vi "ST5 Move Status.vi"(0 "Port COM":refnum<visa-resource-name>, 1 "Facteur Pas":dbl=1500.0, 2 "Facteur Dir":bool, 5 "Delay(s)":i32=40, 9 "Stop Ref":refnum<vi>, 11 "error in":errorcluster, 12 "Pos Ref":refnum<vi>) -> (4 "Port Out":refnum<visa-resource-name>, 6 "CCW Limit":bool, 8 "Alarme":u32, 10 "CW Limit":bool, 14 "Status":T1, 15 "error out":errorcluster)   [LabVIEW 2019]
panel:
  out "Position":dbl
  in  "Stop":bool
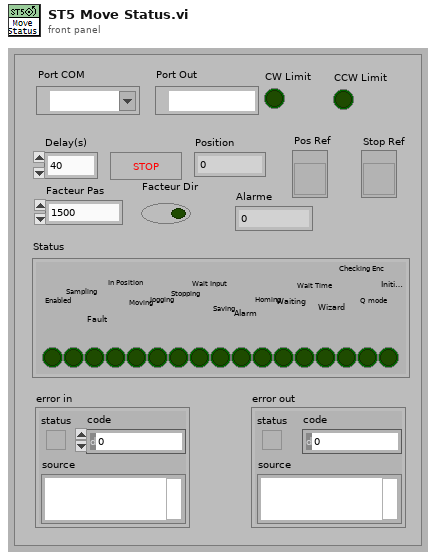
[diagram p1: front panel]
types:
  T1 = cluster{"Enabled":bool, "Sampling":bool, "Fault":bool, "In Position":bool, "Moving":bool, "Jogging":bool, "Stopping":bool, "Wait Input":bool, "Saving":bool, "Alarm":bool, "Homing":bool, "Waiting":bool, "Wait Time":bool, "Wizard":bool, "Checking Enc":bool, "Q mode":bool, "Initializing":bool}
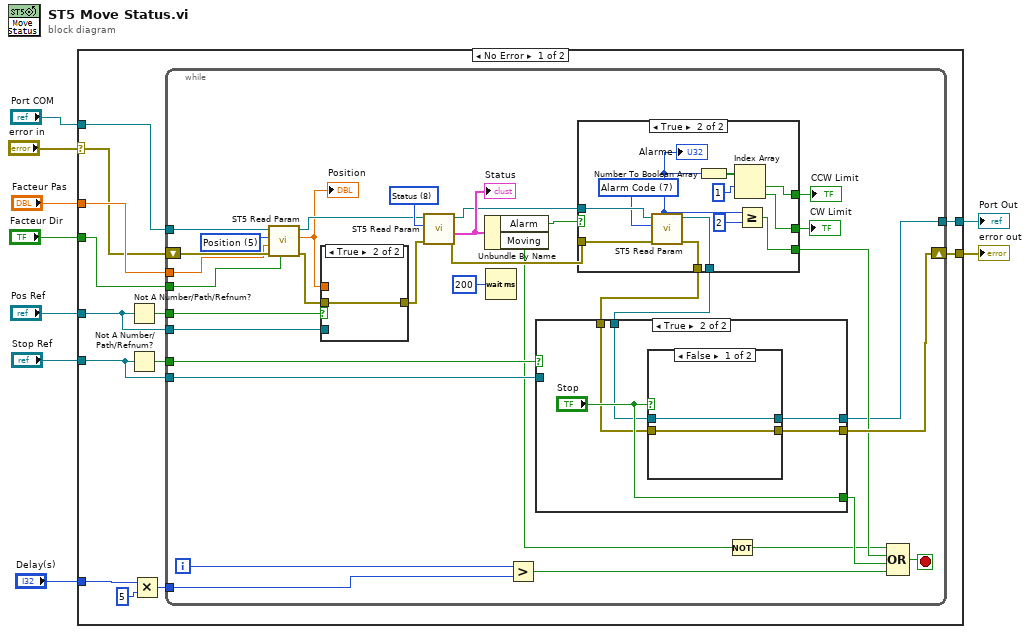
[diagram p0: block diagram]
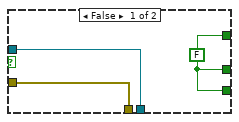
[diagram p2: hidden frame]
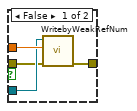
[diagram p3: hidden frame]
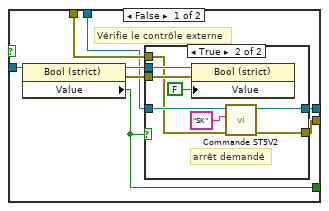
[diagram p4: hidden frame]
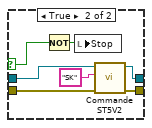
[diagram p6: hidden frame]
diagram:
  n1 = case shown="No Error" "error in" {
    selector: "error in" -> [w12 w109]
    tunnel: [w22 w109] -> w9
    tunnel: "Port COM" -> [w15 w108]
    tunnel: [w21 w108] -> w7
    tunnel: "Delay(s)" -> [w20 _]
    tunnel: "Stop Ref" -> [w16 _]
    tunnel: "Facteur Pas" -> [w14 _]
    tunnel: "Facteur Dir" -> [w13 _]
    tunnel: "Pos Ref" -> [w10 _]
    frame No Error {
      n2 = Not A Number/Path/Refnum?(number/path/refnum=w10) -> (NaN/Path/Refnum?=w11:bool)
      n3 = Not A Number/Path/Refnum?(number/path/refnum=w16) -> (NaN/Path/Refnum?=w17:bool)
      n4 = Multiply(x=w20, y=5) -> (x*y=w18:i32)
      n5 = while {
        tunnel: w15 -> [w46]
        shift-right: [w45] -> w22
        shift-left: w12 -> [w53]
        tunnel: [w25] -> w21
        tunnel: w18 -> [w52]
        tunnel: w17 -> [w50]
        tunnel: w16 -> [w51]
        tunnel: w14 -> [w44]
        tunnel: w13 -> [w40]
        tunnel: w11 -> [w42]
        tunnel: w10 -> [w41]
        i -> [w54]
        stop <- w48 stop-if-true
        w39 = u16 8 items=["All", "Velocity", "Acceleration", "Deceleration", "Max Acceleration", "Position", "Step/Rev", "Alarm Code", "Status"] ("Parameters")
        w43 = u16 5 items=["All", "Velocity", "Acceleration", "Deceleration", "Max Acceleration", "Position", "Step/Rev", "Alarm Code", "Status"] ("Parameters")
        n6 = call <userlib>:"ST5 Read Param.vi"("Facteur Dir"=w40, "error in (no error)"=w53, "Facteur Pas"=w44, "Parameters"=w43, "Port COM"=w46) -> ("error out"=w30:errorcluster, "Position"=w31:dbl, "Port COM Out"=w38:refnum<visa-resource-name>)  [unwired: 4 out]
        "Position" <- w31
        n7 = case shown="True" w42 {
          tunnel: w31 -> [w74 _]
          tunnel: w41 -> [w73 _]
          tunnel: w30 -> [w72 w75]
          tunnel: [w71 w75] -> w29
          frame False {
            n8 = call <userlib>:"WritebyWeakRefNum.vi"("error in"=w72, "Valeur"=w74, "Control Ref"=w73) -> ("error out"=w71:errorcluster)  [unwired: 8 in]
          }
          frame True {
          }
        }
        n9 = call <userlib>:"ST5 Read Param.vi"("error in (no error)"=w29, "Parameters"=w39, "Port COM"=w38) -> ("error out"=w32:errorcluster, "Status"=w34:T1, "Port COM Out"=w27:refnum<visa-resource-name>)  [unwired: 2 in, 4 out]
        "Status" <- w34
        n10 = Unbundle By Name(w34) -> ("Alarm"=w33:bool, "Moving"=w24:bool)
        n11 = Wait (ms)(milliseconds to wait=u32 200) -> ()  [unwired: 1 out]
        n12 = Greater?(x=w54, y=w52) -> (0:w47:bool)
        n13 = case shown="True" w33 {
          tunnel: [w57 w69] -> w37
          tunnel: [w57 w68] -> w36
          tunnel: [w57 w65] -> w35
          tunnel: w32 -> [w58 w64]
          tunnel: [w58 w63] -> w28
          tunnel: w27 -> [w56 w61]
          tunnel: [w56 w60] -> w26
          frame False {
            w57 = FALSE
          }
          frame True {
            w59 = u16 7 items=["All", "Velocity", "Acceleration", "Deceleration", "Max Acceleration", "Position", "Step/Rev", "Alarm Code", "Status"] ("Parameters")
            n14 = call <userlib>:"ST5 Read Param.vi"("error in (no error)"=w64, "Parameters"=w59, "Port COM"=w61) -> ("error out"=w63:errorcluster, "Port COM Out"=w60:refnum<visa-resource-name>, "Alarme"=w62:u32)  [unwired: 2 in, 4 out]
            "Alarme" <- w62
            n15 = Number To Boolean Array(number=w62) -> (Boolean array=w70:bool[])
            n16 = Index Array(array=w70, index #1=1 ("indice")) -> (element #1=w69:bool, element #2=w68:bool)  [unwired: 1 in]
            n17 = Greater Or Equal?(x=w62, y=u32 2) -> (x >= y?=w65:bool)
          }
        }
        "CCW Limit" <- w37
        "CW Limit" <- w36
        n18 = case shown="True" w50 {
          tunnel: w51 -> [w83 _]
          tunnel: [w80 "Stop"] -> w49
          tunnel: w28 -> [w78 w97]
          tunnel: [w79 w96] -> w45
          tunnel: w26 -> [w77 w95]
          tunnel: [w76 w94] -> w25
          frame False {
            # "Vérifie le contrôle externe"
            n19 = property class="Bool (strict)"(reference=w83) -> (reference out=w82:refnum<vi>, error out=w81:errorcluster, "Value"=w80:bool)  [unwired: 1 in]
            n20 = case shown="True" w80 {
              tunnel: w82 -> [_ w93]
              tunnel: w81 -> [_ w92]
              tunnel: w77 -> [w84 w89]
              tunnel: [w85 w88] -> w79
              tunnel: w78 -> [w85 w87]
              tunnel: [w84 w86] -> w76
              frame False {
              }
              frame True {
                # "arrêt demandé"
                n21 = property class="Bool (strict)"(reference=w93, error in=w92, "Value"=FALSE ("Valeur")) -> ()  [unwired: 2 out]
                n22 = call <userlib>:"Commande ST5V2.vi"("error in (no error)"=w87, "Commande"="SK", "Port COM"=w89) -> ("error out"=w88:errorcluster, "Port Out"=w86:refnum<visa-resource-name>)  [unwired: 1 in, 2 out]
              }
            }
          }
          frame True {
            n23 = case shown="False" "Stop" {
              selector: "Stop" -> [_ w106]
              tunnel: w95 -> [w99 w104]
              tunnel: w97 -> [w100 w103]
              tunnel: [w100 w102] -> w96
              tunnel: [w99 w101] -> w94
              frame False {
              }
              frame True {
                n24 = Not(x=w106) -> (.not. x?=w107:bool)
                n25 = local write "Stop"(w107) -> ()
                n26 = call <userlib>:"Commande ST5V2.vi"("error in (no error)"=w103, "Commande"="SK", "Port COM"=w104) -> ("error out"=w102:errorcluster, "Port Out"=w101:refnum<visa-resource-name>)  [unwired: 1 in, 2 out]
              }
            }
          }
        }
        n27 = Not(x=w24) -> (.not. x?=w23:bool)
        n28 = Compound Arithmetic op=OR(w23, w35, w49, w47) -> (w48:bool)
      }
    }
    frame Error {
    }
  }
  "error out" <- w9
  "Port Out" <- w7
